vi "PID Auto Drive.vi"() -> ()   [LabVIEW 2017]
uses:
  PID cluster.ctl
panel:
  in  "Targets":T1
  in  "Tolerances":T2
  in  "Motor Values":T3
  in  "PID Gains":T5
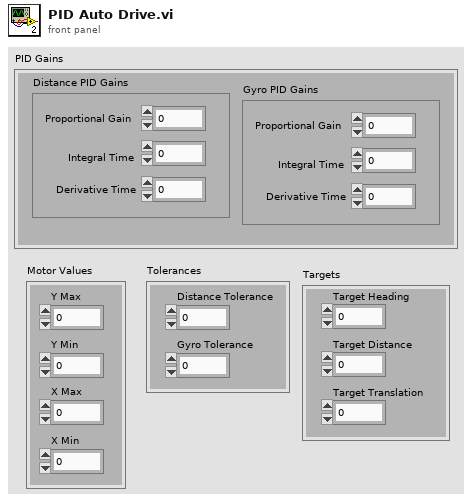
[diagram p1: front panel]
types:
  T1 = cluster{"Target Heading":dbl, "Target Distance":dbl, "Target Translation":dbl}
  T2 = cluster{"Distance Tolerance":dbl, "Gyro Tolerance":dbl}
  T3 = cluster{"Y Max":dbl, "Y Min":dbl, "X Max":dbl, "X Min":dbl}
  T4 = typedef "PID cluster.ctl" = cluster{"Proportional Gain":dbl, "Integral Time":dbl, "Derivative Time":dbl}
  T5 = cluster{"Gyro PID Gains":T4, "Distance PID Gains":T4}
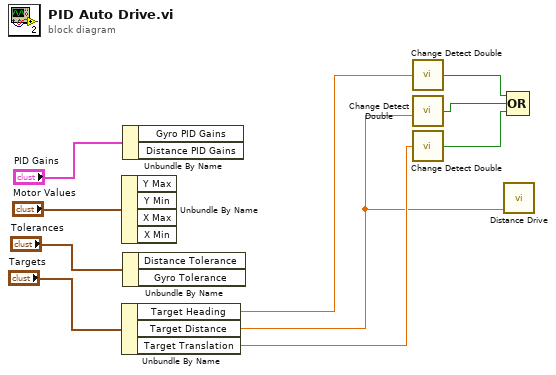
[diagram p0: block diagram]
diagram:
  n1 = Unbundle By Name("Motor Values") -> ()  [unwired: 4 out]
  n2 = Unbundle By Name("Targets") -> ("Target Heading"=w6:dbl, "Target Distance"=w1:dbl, "Target Translation"=w5:dbl)
  n3 = Unbundle By Name("PID Gains") -> ()  [unwired: 2 out]
  n4 = Unbundle By Name("Tolerances") -> ()  [unwired: 2 out]
  n5 = call "Change Detect Double.vi"("In"=w6) -> ("Changed?"=w4:bool)
  n6 = call "Change Detect Double.vi"("In"=w1) -> ("Changed?"=w3:bool)
  n7 = call "Change Detect Double.vi"("In"=w5) -> ("Changed?"=w2:bool)
  n8 = call "Distance Drive.vi"("Numeric 4"=w1) -> ()  [unwired: 11 in]
  n9 = Compound Arithmetic op=OR(w4, w3, w2) -> ()  [unwired: 1 out]
